vi "Goal Distance Calculator.vi"(1 "ResolutionY":dbl, 2 "Theda":dbl, 3 "InArray":dbl[](array[numeric])) -> (0 "DistanceOut":dbl)   [LabVIEW 2012]
panel:
  # "Inputs"
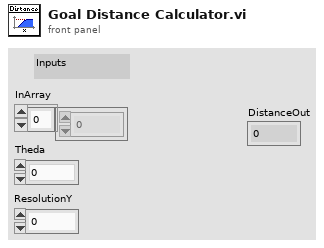
[diagram p1: front panel]
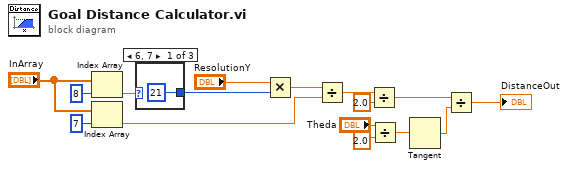
[diagram p0: block diagram]
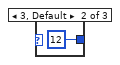
[diagram p2: hidden frame]
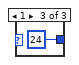
[diagram p3: hidden frame]
diagram:
  n1 = Index Array(array="InArray", index=8) -> (element=w15:dbl)
  n2 = Index Array(array="InArray", index=7) -> (element=w7:dbl)
  n3 = case shown="6, 7" w15 {
    tunnel: [21 12 24] -> w9
    frame 6, 7 {
    }
    frame 3, Default {
    }
    frame 1 {
    }
  }
  n4 = Multiply(x="ResolutionY", y=w9) -> (x*y=w8:dbl)
  n5 = Divide(x=w8, y=w7) -> (x/y=w6:dbl)
  n6 = Divide(x=w6, y=2.0) -> (x/y=w1:dbl)
  n7 = Divide(x="Theda", y=2.0) -> (x/y=w11:dbl)
  n8 = Tangent(1:w11) -> (0:w4:dbl)
  n9 = Divide(x=w1, y=w4) -> (x/y=→"DistanceOut":dbl)
